vi "Untitled 2.vi"() -> ()   [LabVIEW 2010]
panel:
  out "date/time string 2":string
  out "date/time string":string
  out "time stamp":timestamp
  out "current time":timestamp
  out "unsigned 32bit integer":u32
  out "Boolean array":bool[](array[boolean])
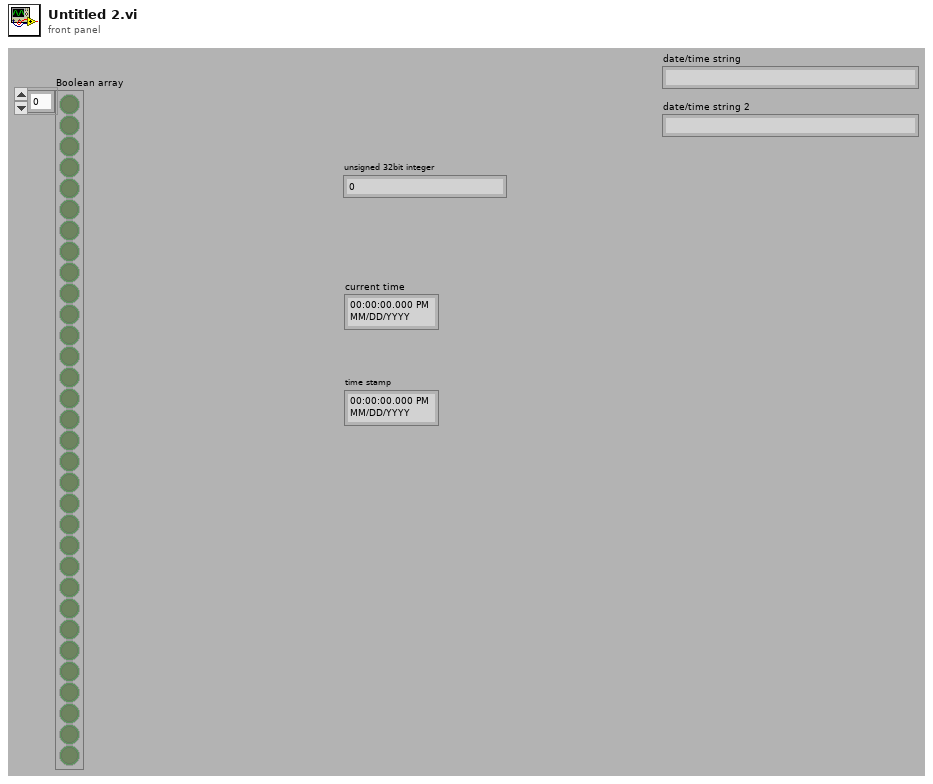
[diagram p1: front panel]
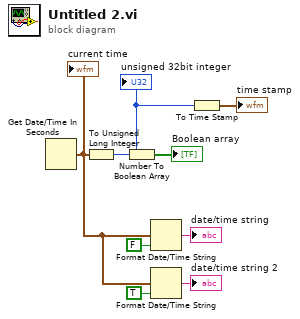
[diagram p0: block diagram]
diagram:
  n1 = Get Date/Time In Seconds() -> (seconds since 1Jan1904=w1:timestamp)
  "current time" <- w1
  n2 = To Unsigned Long Integer(number=w1) -> (unsigned 32bit integer=w7:u32)
  "unsigned 32bit integer" <- w7
  n3 = Number To Boolean Array(number=w7) -> (Boolean array=→"Boolean array":bool[])
  n4 = Format Date/Time String(seconds (now)=w1, UTC format=FALSE) -> (date/time string=→"date/time string":string)  [unwired: 1 in]
  n5 = Format Date/Time String(seconds (now)=w1, UTC format=TRUE) -> (date/time string=→"date/time string 2":string)  [unwired: 1 in]
  n6 = To Time Stamp(1:w7) -> (0:→"time stamp":timestamp)
